vi "Point Value Map DEBUG ReadAllPoints.vi"() -> ()   [LabVIEW 2017]
uses:
  <vilib>/addons/PointValueMap/controls/Point.ctl
  <vilib>/addons/PointValueMap/controls/DataTypes.ctl
  <vilib>/addons/PointValueMap/PointValueMap.lvlib
panel:
  out "All Map Names":string[](array[string])
  out "Points":T1[](array[typedef])
  out "Names":string[](array[string])
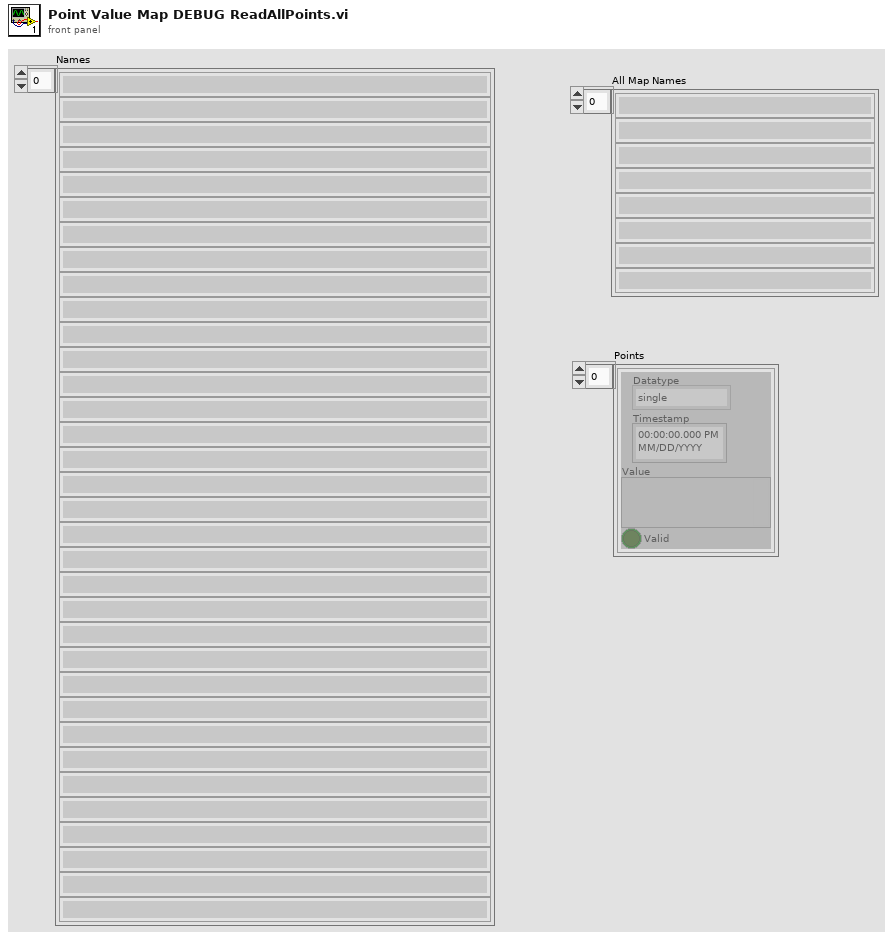
[diagram p1: front panel]
types:
  T1 = typedef "PointValueMap.lvlib/Point.ctl" = cluster{"Datatype":T2, "Timestamp":timestamp, "Value":variant, "Valid":bool}
  T2 = typedef "PointValueMap.lvlib/DataTypes.ctl" = enum16{"single", "double", "i32", "string", "variant"}
  T3 = typedef "PointValueMap.lvlib/PointMap.ctl" = refnum<data-value>
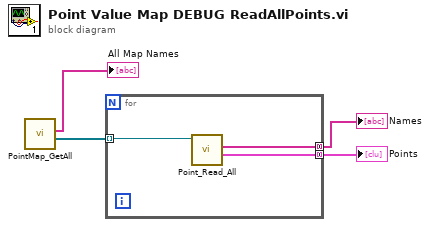
[diagram p0: block diagram]
diagram:
  n1 = call <vilib>:"PointMap_GetAll.vi"() -> ("All Maps"=w4:T3[], "All Map Names"=→"All Map Names":string[])  [unwired: 9 in, 1 out]
  n2 = for {
    tunnel: w4 -> [w7] mode=indexing
    tunnel: [w6] -> w3 mode=concatenating
    tunnel: [w5] -> w2 mode=concatenating
    n3 = call <vilib>:"Point_Read_All.vi"("Map"=w7) -> ("Points"=w5:T1[], "Names"=w6:string[])  [unwired: 7 in, 2 out]
  }
  "Names" <- w3
  "Points" <- w2
